vi "Generate Random Bits.vi"(3 "markov":dbl[][](array[numeric]), 4 "symbol map":cdb[](array[numeric]) format="%.3f", 5 "LastValue":i32, 6 "Number of Bits":i32) -> (0 "error out":errorcluster, 1 "NextValue":i32, 2 "output":cdb[](array[numeric]))   [LabVIEW 2014]
uses:
  <vilib>/addons/Modulation/Digital/General/MT Generate Bits (Galois, PN Order).vi
  <vilib>/addons/Modulation/Digital/Support/Common/Validators/mod_Generate Bits Validate.vi
  <vilib>/addons/Modulation/Analog/support/mod_Set Error Source.vi
  <vilib>/addons/Modulation/Digital/General/subVIs/mod_Generate Bits PN Sequence.vi
  <vilib>/addons/Modulation/Digital/General/MT Map Bits to QAM Symbols.vi
  <vilib>/addons/Modulation/niDMT.lvlib
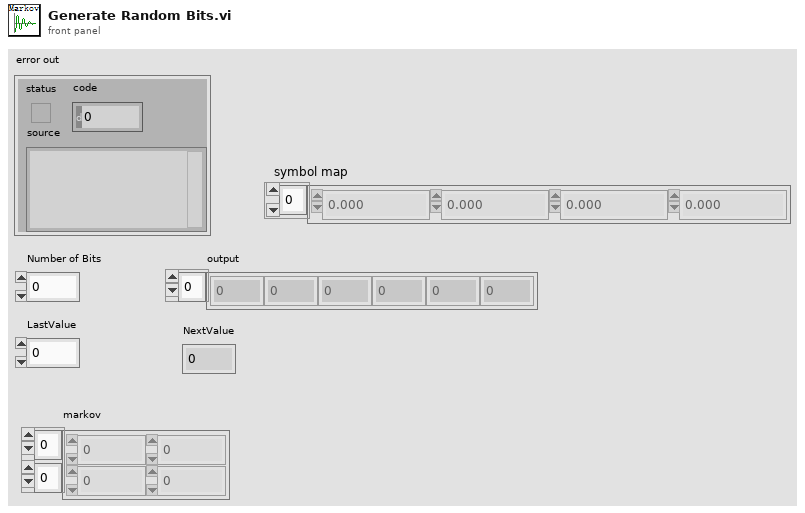
[diagram p1: front panel]
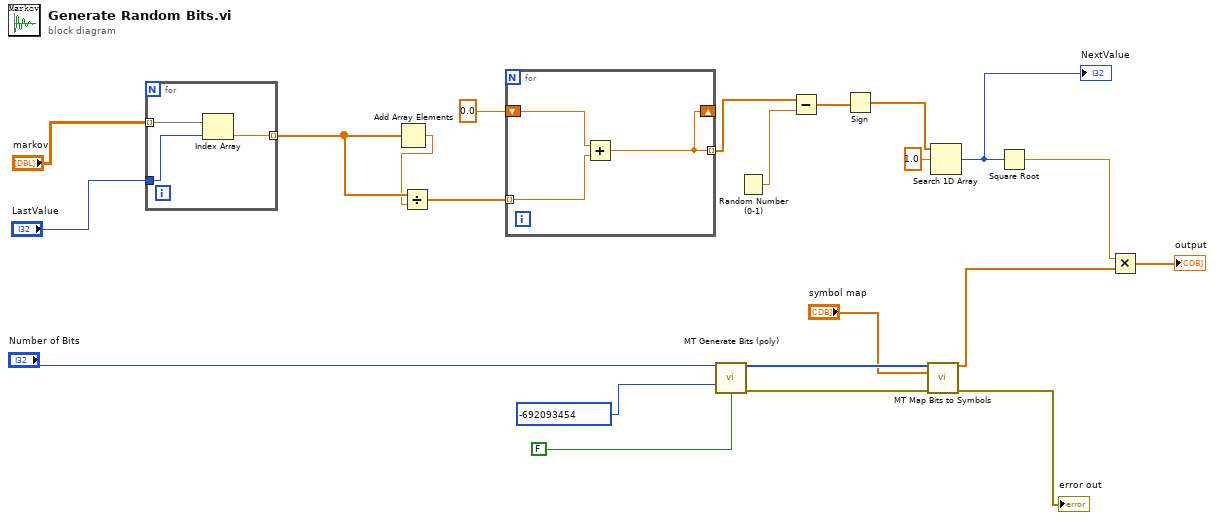
[diagram p0: block diagram]
diagram:
  n1 = for {
    tunnel: "markov" -> [w25] mode=indexing
    tunnel: "LastValue" -> [w24]
    tunnel: [w23] -> w17 mode=indexing
    n2 = Index Array(array=w25, index=w24) -> (element=w23:dbl)
  }
  n3 = Add Array Elements(numeric array=w17) -> (sum=w16:dbl)
  n4 = Divide(x=w17, y=w16) -> (x/y=w15:dbl[])
  n5 = for {
    tunnel: w15 -> [w28] mode=indexing
    shift-right: [w26] -> _
    shift-left: 0.0 -> [w27]
    tunnel: [w26] -> w13 mode=indexing
    n6 = Add(x=w27, y=w28) -> (x+y=w26:dbl)
  }
  n7 = call-poly <vilib>:"MT Generate Bits (poly).vi"("total bits (128)"="Number of Bits", "seed in (0xD6BF7DF2)"=-692093454, "reset? (T)"=FALSE) -> ("output bit stream"=w5:i8[], "error out"=w6:errorcluster)  [unwired: 10 in, 1 out]
  n8 = Random Number (0-1)() -> (number: 0 to 1=w12:dbl)
  n9 = Subtract(x=w13, y=w12) -> (x-y=w11:dbl[])
  n10 = Sign(1:w11) -> (0:w10:dbl[])
  n11 = call-poly <vilib>:"MT Map Bits to Symbols.vi"("input bit stream"=w5, "symbol map"="symbol map", "error in (no error)"=w6) -> ("symbols"=w4:cdb[], "error out"=→"error out":errorcluster)  [unwired: 11 in]
  n12 = Search 1D Array(1D array=w10, element=1.0) -> (index of element=w8:i32)  [unwired: 1 in]
  "NextValue" <- w8
  n13 = Square Root(x=w8) -> (sqrt(x)=w7:dbl)
  n14 = Multiply(x=w7, y=w4) -> (x*y=→"output":cdb[])
